vi "2526 Disconnect.vi"(8 "error in (no error)":errorcluster, 9 "Index":i32, 10 "2525 Scan List Channels":string[](array[string]), 11 "IVI Refnum in":refnum<k15>) -> (0 "error out":errorcluster, 3 "IVI Refnum out":refnum<k15>)   [LabVIEW 2019, in "SupportVIs.lvlib"]
uses:
  SupportVIs.lvlib
  <instrlib>/niSwitch/niSwitch.llb/niSwitch Disconnect Channels (Single).vi
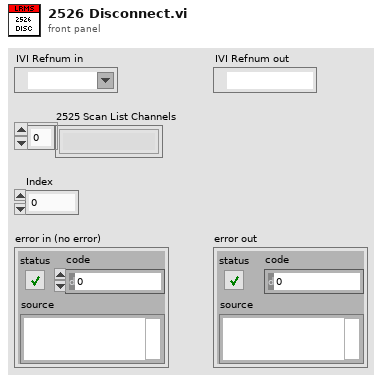
[diagram p1: front panel]
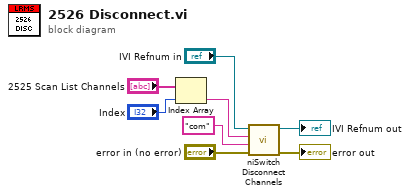
[diagram p0: block diagram]
diagram:
  n1 = Index Array(array="2525 Scan List Channels", index="Index") -> (element=w1:string)
  n2 = call-poly <instrlib>:"niSwitch Disconnect Channels.vi"("error in (no error)"="error in (no error)", "channel 2"="com", "channel 1"=w1, "instrument handle"="IVI Refnum in") -> ("error out"=→"error out":errorcluster, "instrument handle out"=→"IVI Refnum out":refnum<k15>)  [unwired: 6 in]
